vi "SDG X Series Arbitrary Waveform.vi"() -> ()   [LabVIEW 2015]
doc: "This example shows how to create then configure an arbitrary waveform."
uses:
  Instance           1 56Saved   Template - Function Generator Arbitrary Waveform .vi
  Instance           2 56Saved   Template - Function Generator Arbitrary Waveform .vi
  <instrlib>/SDG X Series/SDG X Series.lvlib
panel:
  in  "VISA resource name":refnum<visa-resource-name>
  in  "DC Offset (0.00 V)":dbl
  in  "Frequency (1000 Hz)":dbl=1000.0 format="%#.6g"
  in  "Amplitude (1.0 Vpp)":dbl=1.0 format="%#.3f"
  in  "Channel (1:Channel 1)":i32(ring)=1 items=["Channel 1"=1, "Channel 2"=2]
  in  "Arbitrary Waveform Name":string="ARB1"
  # "(c) 2017 SIGLENT TECHNOLOGIES CO.,LTD. ALL RIGHTS RESERVED."
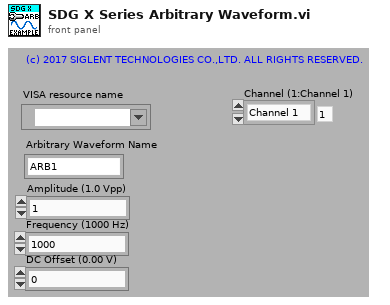
[diagram p1: front panel]
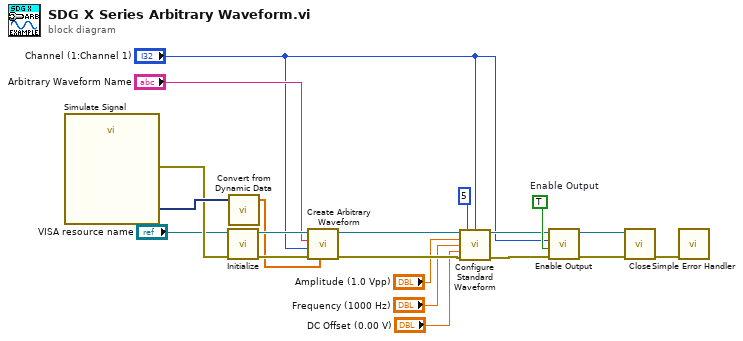
[diagram p0: block diagram]
diagram:
  w12 = TRUE  # Enable Output
  n1 = call "Simulate Signal"() -> ("正弦"=w20:dynamicdata, "error out"=w19:errorcluster)  [unwired: 14 in]
  n2 = call <instrlib>:"Initialize.vi"("error in (no error)"=w19, "VISA resource name"="VISA resource name") -> ("error out"=w15:errorcluster, "VISA resource name out"=w14:refnum<visa-resource-name>)  [unwired: 8 in]
  n3 = call "Convert from Dynamic Data"("Dynamic Data Type"=w20) -> ("Array"=w3:dbl[])  [unwired: 3 in]
  n4 = call <instrlib>:"Create Arbitrary Waveform.vi"("Arbitrary Numeric Waveform Data"=w3, "error in (no error)"=w15, "Select Channel (1:Channel 1)"="Channel (1:Channel 1)", "Waveform Name (\"wave1\")"="Arbitrary Waveform Name", "VISA resource name"=w14) -> ("error out"=w9:errorcluster, "VISA resource name out"=w11:refnum<visa-resource-name>)  [unwired: 5 in]
  n5 = call <instrlib>:"Configure Standard Waveform.vi"("VISA resource name"=w11, "Waveform Function (0: Sine)"=5, "Channel (1:Channel 1)"="Channel (1:Channel 1)", "Amplitude (1.0 Vpp)"="Amplitude (1.0 Vpp)", "Frequency (1000 Hz)"="Frequency (1000 Hz)", "DC Offset (0.00 V)"="DC Offset (0.00 V)", "error in (no error)"=w9) -> ("VISA resource name out"=w10:refnum<visa-resource-name>, "error out"=w8:errorcluster)  [unwired: 7 in]
  n6 = call <instrlib>:"Enable Output.vi"("error in (no error)"=w8, "Enable Output (T: Enable)"=w12, "Channel (1:Channel 1)"="Channel (1:Channel 1)", "VISA resource name"=w10) -> ("error out"=w17:errorcluster, "VISA resource name out"=w16:refnum<visa-resource-name>)  [unwired: 6 in]
  n7 = call <instrlib>:"Close.vi"("error in (no error)"=w17, "VISA resource name"=w16) -> ("error out"=w18:errorcluster)  [unwired: 9 in]
  n8 = call <vilib>:"Simple Error Handler.vi"("error in (no error)"=w18) -> ()  [unwired: 4 in, 5 out]
